vi "Meter Detection ActionVIOnSave.vi"(8 "error in (no error)":errorcluster, 11 "Device Item Ref in":T1 format="%.0x") -> (0 "error out":errorcluster, 3 "Device Item Ref out":T1 format="%.0x")   [LabVIEW 2011, in "Meter Detection Custom Device.lvlib"]
uses:
  Meter Detection Custom Device.lvlib
  <vilib>/NI Veristand/Custom Device API/Custom Device Item Ref.ctl
  <vilib>/vision/NI_Vision_Development_Module.lvlib
  <vilib>/NI Veristand/Custom Device API/Custom Device API.lvlib
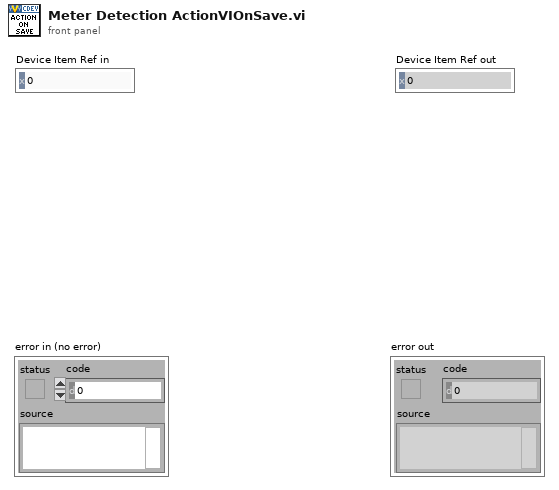
[diagram p1: front panel]
types:
  T1 = typedef "Custom Device API.lvlib/Custom Device Item Ref.ctl" = u64
  T2 = cluster{"Global Rectangle":i32[], "Contours":cluster{"Contour Type":u32, "ROI Type":u32, "Points":i32[]}[]}
  T3 = cluster{"Global Rectangle":i32[], "Contours":cluster{"Contour Type":u32, "ROI Type":u32, "Points":i32[]}[]}[]
  T4 = typedef "ROI Descriptor" = cluster{"Global Rectangle":i32[], "Contours":cluster{"ID":enum32{"External", "Internal"}, "Type":u32, "Coordinates":i32[]}[]}
  T5 = typedef "IMAQ Image.ctl" = refnum<image>
  T6 = typedef "Custom Device API.lvlib/Custom Device Item Info.ctl" = cluster{"Name":string, "Is Channel":bool, "GUID":string}
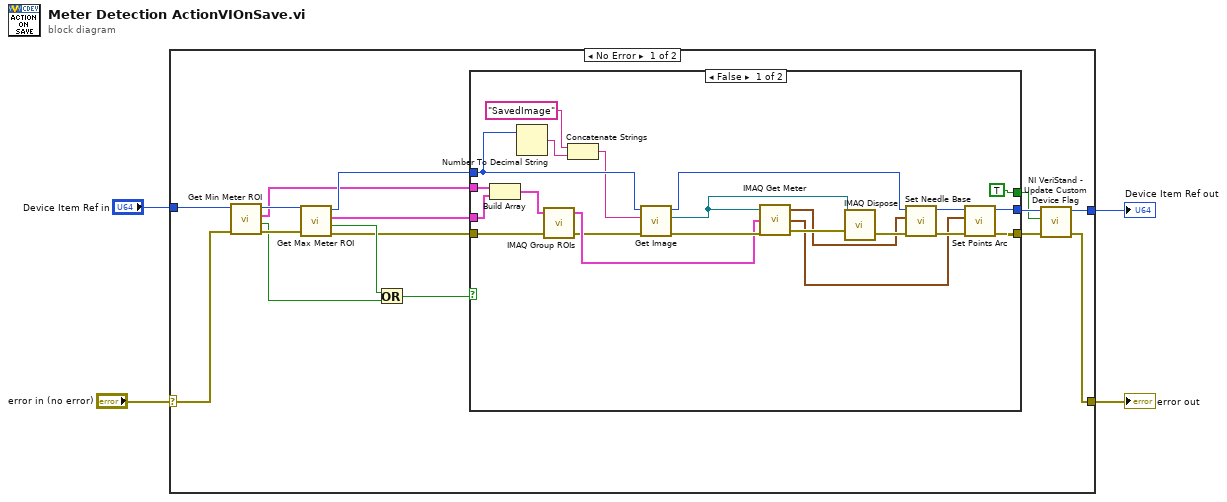
[diagram p0: block diagram]
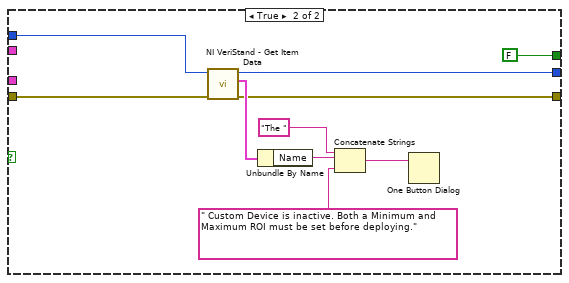
[diagram p2: hidden frame]
diagram:
  n1 = case shown="No Error" "error in (no error)" {
    selector: "error in (no error)" -> [w20 w54]
    tunnel: [w10 w54] -> w3
    tunnel: "Device Item Ref in" -> [w9 w53]
    tunnel: [w11 w53] -> w1
    frame No Error {
      n2 = call "Get Min Meter ROI.vi"("error in (no error)"=w20, "Item Ref in"=w9) -> ("error out"=w19:errorcluster, "empty?"=w17:bool, "Max Gauge ROI"=w7:T2, "Item Ref out"=w18:T1)  [unwired: 6 in]
      n3 = call "Get Max Meter ROI.vi"("error in (no error)"=w19, "Item Ref in"=w18) -> ("error out"=w5:errorcluster, "empty?"=w16:bool, "Max Gauge ROI"=w6:T2, "Item Ref out"=w8:T1)  [unwired: 6 in]
      n4 = Or(x=w16, y=w17) -> (x .or. y?=w15:bool)
      n5 = case shown="False" w15 {
        tunnel: [w37 w46] -> w14
        tunnel: [w36 w45] -> w13
        tunnel: w5 -> [w22 w51]
        tunnel: w8 -> [w29 w52]
        tunnel: [TRUE ("Is Custom Device Active?") FALSE ("Is Custom Device Active?")] -> w12
        tunnel: w7 -> [w26 _]
        tunnel: w6 -> [w25 _]
        frame False {
          n6 = Build Array(w26, w25) -> (w24:T3)
          n7 = Number To Decimal String(number=w29) -> (decimal integer string=w30:string)  [unwired: 1 in]
          n8 = call "IMAQ Group ROIs"("error in (no error)"=w22, "ROI Descriptors"=w24) -> ("error out"=w21:errorcluster, "ROI Descriptor out"=w23:T4)  [unwired: 2 in]
          n9 = Concatenate Strings("SavedImage" ("Image Name"), w30) -> (w27:string)
          n10 = call "Get Image.vi"("error in (no error)"=w21, "Image Name"=w27, "Item Ref out out"=w29) -> ("error out"=w32:errorcluster, "Image out"=w31:T5, "Item Ref out"=w33:T1)  [unwired: 5 in, 1 out]
          n11 = call "IMAQ Get Meter"("Image"=w31, "ROI Descriptor"=w23, "error in (no error)"=w32) -> ("Needle Base"=w35:cluster{"X":sgl, "Y":sgl}, "Points Arc"=w39:cluster{"X":sgl, "Y":sgl}[], "error out"=w42:errorcluster)  [unwired: 4 in]
          n12 = call "IMAQ Dispose"("Image"=w31, "error in (no error)"=w42) -> ("error out"=w41:errorcluster)  [unwired: 4 in]
          n13 = call "Set Needle Base.vi"("error in (no error)"=w41, "Needle Base"=w35, "Item Ref in"=w33) -> ("error out"=w40:errorcluster, "Item Ref out"=w38:T1)  [unwired: 7 in]
          n14 = call "Set Points Arc.vi"("error in (no error)"=w40, "Points Arc"=w39, "Item Ref in"=w38) -> ("error out"=w37:errorcluster, "Item Ref out"=w36:T1)  [unwired: 7 in]
        }
        frame True {
          n15 = call <vilib>:"NI VeriStand - Get Item Data.vi"("error in (no error)"=w51, "Item Ref in"=w52) -> ("error out"=w46:errorcluster, "Item Info"=w50:T6, "Item Ref out"=w45:T1)  [unwired: 6 in, 1 out]
          n16 = Unbundle By Name(w50) -> ("Name"=w49:string)
          n17 = Concatenate Strings("The " ("string"), w49, " Custom Device is inactive. Both a Minimum and Maximum ROI must be set before deploying." ("message")) -> (w47:string)
          n18 = One Button Dialog(message=w47) -> ()  [unwired: 1 in, 1 out]
        }
      }
      n19 = call <vilib>:"NI VeriStand - Update Custom Device Flag.vi"("error in (no error)"=w14, "Is Custom Device Active?"=w12, "Device Ref in"=w13) -> ("error out"=w10:errorcluster, "Device Ref out"=w11:T1)  [unwired: 7 in]
    }
    frame Error {
    }
  }
  "error out" <- w3
  "Device Item Ref out" <- w1
